vi "dianyacaiji-5.5.vi"() -> (1 "测量电压":dbl)   [LabVIEW 2015]
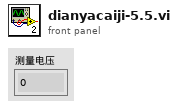
[diagram p1: front panel]
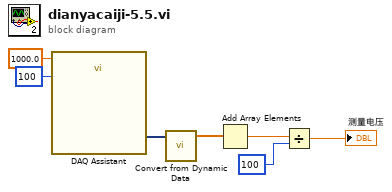
[diagram p0: block diagram]
diagram:
  n1 = call "DAQ Assistant"("rate"=1000.0, "number of samples"=100) -> ("data"=w5:dynamicdata)  [unwired: 15 in, 2 out]
  n2 = call "Convert from Dynamic Data"("Dynamic Data Type"=w5) -> ("Array"=w4:dbl[])  [unwired: 3 in]
  n3 = Add Array Elements(numeric array=w4) -> (sum=w3:dbl)
  n4 = Divide(x=w3, y=i8 100) -> (x/y=→"测量电压":dbl)
